vi "Agilent VNA Read IFBW.vi"(6 "Channel":i8=1 min=1 max=99 step=1, 7 "Agilent VNA":T1, 8 "error in (no error)":errorcluster, 11 "VISA Resource Name":refnum<visa-resource-name>) -> (0 "error out":errorcluster, 2 "IFBW, Hz":dbl=3000.0, 3 "dup VISA Resource Name":refnum<visa-resource-name>)   [LabVIEW 2011]
doc: "This Vi for the HP8753B Network Analyzer is used to set averaging, smoothing, and the IF bandwidth."
uses:
  TypeDefs/Agilent VNA Instrument Info.ctl
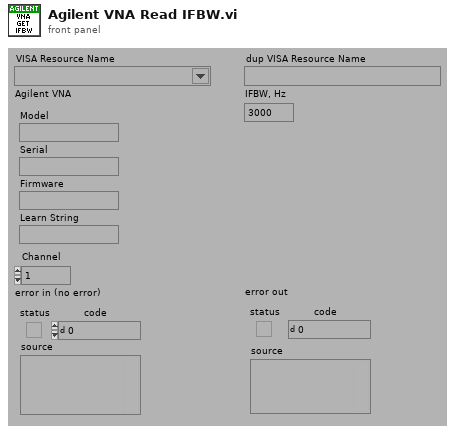
[diagram p1: front panel]
types:
  T1 = typedef "Agilent VNA Instrument Info.ctl" = cluster{"Model":string, "Serial":string, "Firmware":string, "Learn String":string}
  T2 = typedef "Agilent VNA Model.ctl" = enum16{"Not Supported", "8510X", "8719X", "8720X", "8722X", "8753X", "ENA", "PNA", "Field Fox"}
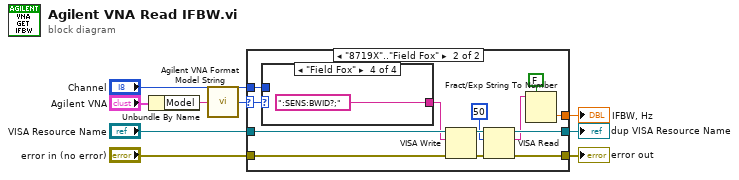
[diagram p0: block diagram]
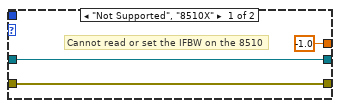
[diagram p2: hidden frame]
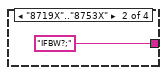
[diagram p4: hidden frame]
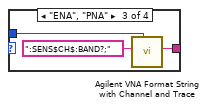
[diagram p5: hidden frame]
diagram:
  n1 = Unbundle By Name("Agilent VNA") -> ("Model"=w1:string)
  n2 = call "Agilent VNA Format Model String.vi"("Model"=w1) -> ("Model"=w3:T2)
  n3 = case shown="\"8719X\"..\"Field Fox\"" w3 {
    selector: w3 -> [_ w13]
    tunnel: "VISA Resource Name" -> [w11 w25]
    tunnel: "error in (no error)" -> [w12 w24]
    tunnel: [w11 w22] -> w7
    tunnel: [w12 w18] -> w6
    tunnel: [-1.0 w16] -> w5
    tunnel: "Channel" -> [_ w14]
    frame "Not Supported", "8510X" {
      # "Cannot read or set the IFBW on the 8510"
    }
    frame "8719X".."Field Fox" {
      n4 = case shown="\"Field Fox\"" w13 {
        tunnel: [_ "IFBW?;" w28 ":SENS:BWID?;"] -> w15
        tunnel: w14 -> [_ _ w27 _]
        frame "Not Supported", "8510X" {
        }
        frame "8719X".."8753X" {
        }
        frame "ENA", "PNA" {
          n5 = call "Agilent VNA Format String with Channel and Trace.vi"("Channel"=w27, "String"=":SENS$CH$:BAND?;") -> ("String Out"=w28:string)  [unwired: 1 in, 6 out]
        }
        frame "Field Fox" {
        }
      }
      n6 = VISA Write(VISA resource name=w25, write buffer=w15, error in (no error)=w24) -> (VISA resource name out=w23:refnum<visa-resource-name>, error out=w19:errorcluster)  [unwired: 1 out]
      n7 = VISA Read(VISA resource name=w23, byte count=u32 50, error in (no error)=w19) -> (VISA resource name out=w22:refnum<visa-resource-name>, read buffer=w17:string, error out=w18:errorcluster)  [unwired: 1 out]
      n8 = Fract/Exp String To Number(use system decimal point (T)=FALSE, string=w17) -> (number=w16:dbl)  [unwired: 3 out]
    }
  }
  "error out" <- w6
  "dup VISA Resource Name" <- w7
  "IFBW, Hz" <- w5
